vi "NewNearestNeighbor.vi"(4 "w":dbl=inf format="%#_13g", 6 "index":i32, 9 "p":dbl[](array[numeric]), 10 "q":dbl[](array[numeric]), 11 "KD-Tree":T1) -> (2 "Nearest":dbl[](array[numeric]))   [LabVIEW 2018]
uses:
  KD-Tree.ctl
  Node.ctl
  <vilib>/Analysis/_algsub.llb/Real Vector Norm.vi
  <vilib>/Analysis/NI_AALPro.lvlib
panel:
  out "Elapsed Time (s)":dbl
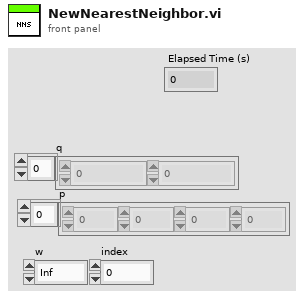
[diagram p1: front panel]
types:
  T1 = typedef "KD-Tree.ctl" = T2[]
  T2 = typedef "Node.ctl" = cluster{"axis":enum16{"null", "x", "y"}, "value":dbl, "left":dbl, "right":dbl, "Point":dbl[]}
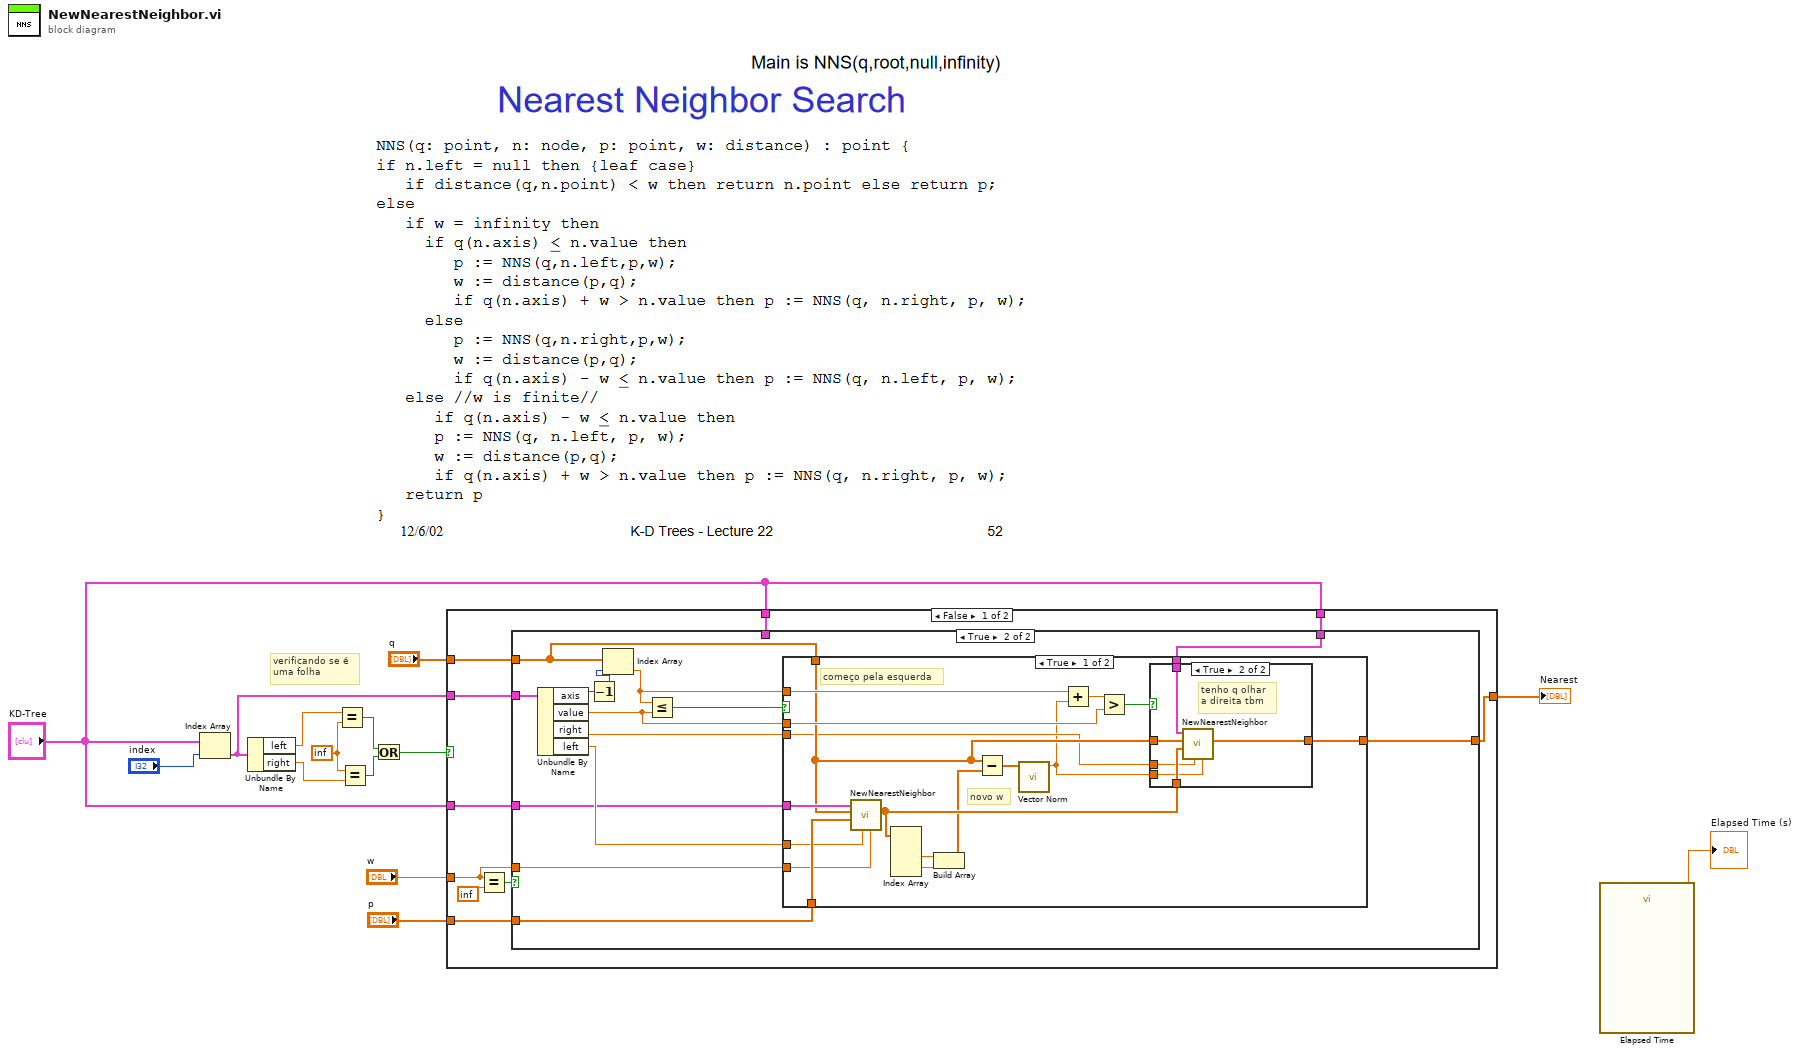
[diagram p0: block diagram]
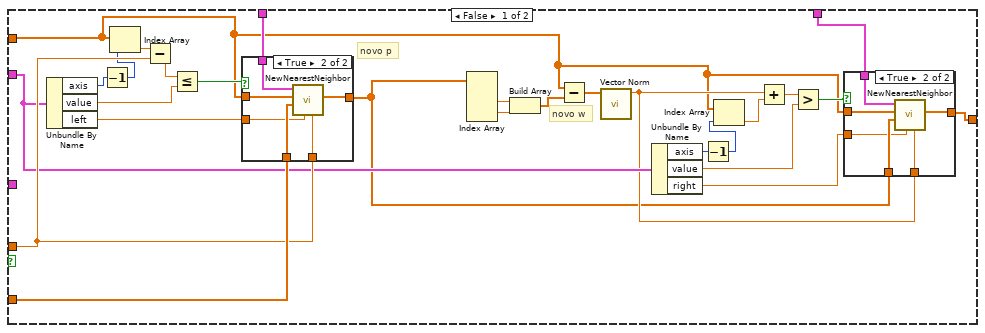
[diagram p2: hidden frame]
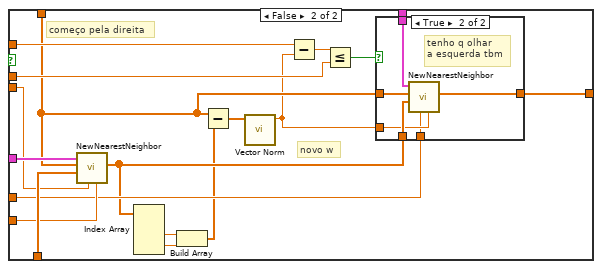
[diagram p6: hidden frame]
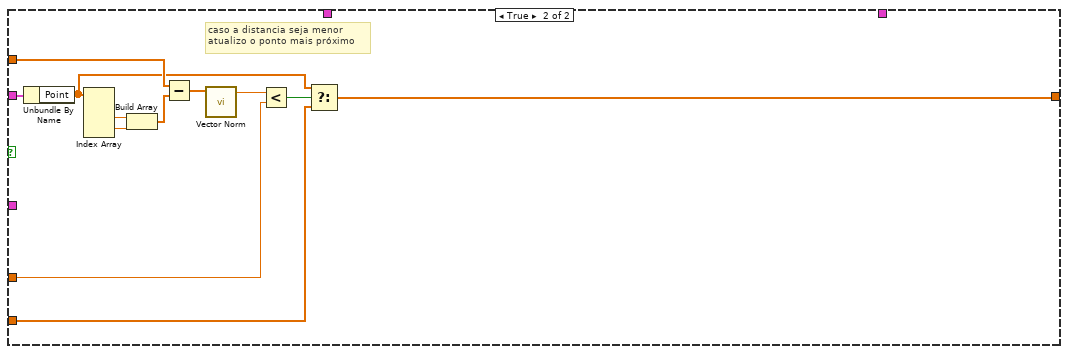
[diagram p8: hidden frame]
diagram:
  w13 = inf
  # "verificando se é \numa folha"
  n1 = Index Array(array="KD-Tree", index="index") -> (element=w7:T2)
  n2 = Unbundle By Name(w7) -> ("left"=w11:dbl, "right"=w12:dbl)
  n3 = Equal?(x=w11, y=w13) -> (x = y?=w9:bool)
  n4 = Equal?(x=w13, y=w12) -> (x = y?=w10:bool)
  n5 = Or(x=w9, y=w10) -> (x .or. y?=w8:bool)
  n6 = case shown="False" w8 {
    tunnel: w7 -> [w22 w141]
    tunnel: "q" -> [w21 w138]
    tunnel: "w" -> [w18 w135]
    tunnel: "p" -> [w19 w133]
    tunnel: [w16 w132] -> w3
    tunnel: "KD-Tree" -> [w20 _]
    tunnel: "KD-Tree" -> [w17 _]
    tunnel: "KD-Tree" -> [w15 _]
    frame False {
      n7 = Equal?(x=w18, y=inf) -> (x = y?=w24:bool)
      n8 = case shown="True" w24 {
        tunnel: w22 -> [w42 w79]
        tunnel: w21 -> [w33 w77]
        tunnel: w20 -> [_ w70]
        tunnel: w19 -> [w46 w76]
        tunnel: w18 -> [w44 w75]
        tunnel: w17 -> [w34 w69]
        tunnel: [w37 w68] -> w16
        tunnel: w15 -> [w47 _]
        frame False {
          # "novo p"
          # "novo w"
          n9 = Unbundle By Name(w42) -> ("axis"=w32:enum16{"null", "x", "y"}, "value"=w49:dbl, "left"=w45:dbl)
          n10 = Decrement(x=w32) -> (x-1=w31:enum16{"null", "x", "y"})
          n11 = Index Array(array=w33, index=w31) -> (element=w51:dbl)
          n12 = Subtract(x=w51, y=w44) -> (x-y=w50:dbl)
          n13 = Less Or Equal?(x=w50, y=w49) -> (x <= y?=w48:bool)
          n14 = case shown="True" w48 {
            tunnel: w47 -> [_ w65]
            tunnel: w33 -> [_ w64]
            tunnel: w46 -> [w59 w63]
            tunnel: w45 -> [_ w62]
            tunnel: w44 -> [_ w61]
            tunnel: [w59 w60] -> w26
            frame False {
            }
            frame True {
              n15 = call "NewNearestNeighbor.vi"("w"=w61, "index"=w62, "p"=w63, "q"=w64, "KD-Tree"=w65) -> ("Nearest"=w60:dbl[])  [unwired: 6 in]
            }
          }
          n16 = Index Array(array=w26) -> (element #2=w28:dbl, element #3=w27:dbl)  [unwired: 4 in, 2 out]
          n17 = Build Array(w28, w27) -> (w25:dbl[])
          n18 = Subtract(x=w33, y=w25) -> (x-y=w43:dbl[])
          n19 = call-poly <vilib>:"Vector Norm.vi"("Input Vector"=w43) -> ("norm"=w35:dbl)  [unwired: 9 in, 1 out]
          n20 = Unbundle By Name(w42) -> ("axis"=w30:enum16{"null", "x", "y"}, "value"=w39:dbl, "right"=w36:dbl)
          n21 = Decrement(x=w30) -> (x-1=w29:enum16{"null", "x", "y"})
          n22 = Index Array(array=w33, index=w29) -> (element=w41:dbl)
          n23 = Add(x=w35, y=w41) -> (x+y=w40:dbl)
          n24 = Greater?(x=w40, y=w39) -> (0:w38:bool)
          n25 = case shown="True" w38 {
            tunnel: w34 -> [_ w58]
            tunnel: w33 -> [_ w57]
            tunnel: w26 -> [w52 w56]
            tunnel: w36 -> [_ w55]
            tunnel: w35 -> [_ w54]
            tunnel: [w52 w53] -> w37
            frame False {
            }
            frame True {
              n26 = call "NewNearestNeighbor.vi"("w"=w54, "index"=w55, "p"=w56, "q"=w57, "KD-Tree"=w58) -> ("Nearest"=w53:dbl[])  [unwired: 6 in]
            }
          }
        }
        frame True {
          n27 = Unbundle By Name(w79) -> ("axis"=w67:enum16{"null", "x", "y"}, "value"=w71:dbl, "right"=w73:dbl, "left"=w74:dbl)
          n28 = Decrement(x=w67) -> (x-1=w66:enum16{"null", "x", "y"})
          n29 = Index Array(array=w77, index=w66) -> (element=w72:dbl)
          n30 = Less Or Equal?(x=w72, y=w71) -> (x <= y?=w78:bool)
          n31 = case shown="True" w78 {
            tunnel: w70 -> [w89 w115]
            tunnel: w77 -> [w87 w113]
            tunnel: w76 -> [w97 w122]
            tunnel: w74 -> [w96 w109]
            tunnel: w75 -> [w95 w121]
            tunnel: w73 -> [w86 w110]
            tunnel: w72 -> [w93 w119]
            tunnel: w71 -> [w91 w117]
            tunnel: w69 -> [w88 w114]
            tunnel: [w84 w111] -> w68
            frame True {
              # "novo w"
              # "começo pela esquerda"
              n32 = call "NewNearestNeighbor.vi"("w"=w95, "index"=w96, "p"=w97, "q"=w87, "KD-Tree"=w89) -> ("Nearest"=w81:dbl[])  [unwired: 6 in]
              n33 = Index Array(array=w81) -> (element #2=w83:dbl, element #3=w82:dbl)  [unwired: 4 in, 2 out]
              n34 = Build Array(w83, w82) -> (w80:dbl[])
              n35 = Subtract(x=w87, y=w80) -> (x-y=w94:dbl[])
              n36 = call-poly <vilib>:"Vector Norm.vi"("Input Vector"=w94) -> ("norm"=w85:dbl)  [unwired: 9 in, 1 out]
              n37 = Add(x=w93, y=w85) -> (x+y=w92:dbl)
              n38 = Greater?(x=w92, y=w91) -> (0:w90:bool)
              n39 = case shown="True" w90 {
                tunnel: w88 -> [_ w104]
                tunnel: w87 -> [_ w103]
                tunnel: w81 -> [w98 w102]
                tunnel: w86 -> [_ w101]
                tunnel: w85 -> [_ w100]
                tunnel: [w98 w99] -> w84
                frame False {
                  # "n é necessário \nolhar a direita"
                }
                frame True {
                  # "tenho q olhar \na direita tbm"
                  n40 = call "NewNearestNeighbor.vi"("w"=w100, "index"=w101, "p"=w102, "q"=w103, "KD-Tree"=w104) -> ("Nearest"=w99:dbl[])  [unwired: 6 in]
                }
              }
            }
            frame False {
              # "novo w"
              # "começo pela direita"
              n41 = call "NewNearestNeighbor.vi"("w"=w121, "index"=w110, "p"=w122, "q"=w113, "KD-Tree"=w115) -> ("Nearest"=w106:dbl[])  [unwired: 6 in]
              n42 = Index Array(array=w106) -> (element #2=w108:dbl, element #3=w107:dbl)  [unwired: 4 in, 2 out]
              n43 = Build Array(w108, w107) -> (w105:dbl[])
              n44 = Subtract(x=w113, y=w105) -> (x-y=w120:dbl[])
              n45 = call-poly <vilib>:"Vector Norm.vi"("Input Vector"=w120) -> ("norm"=w112:dbl)  [unwired: 9 in, 1 out]
              n46 = Subtract(x=w119, y=w112) -> (x-y=w118:dbl)
              n47 = Less Or Equal?(x=w118, y=w117) -> (x <= y?=w116:bool)
              n48 = case shown="True" w116 {
                tunnel: w114 -> [_ w129]
                tunnel: w113 -> [_ w128]
                tunnel: w106 -> [w123 w127]
                tunnel: w112 -> [_ w126]
                tunnel: [w123 w125] -> w111
                tunnel: w109 -> [_ w124]
                frame False {
                  # "n é necessário \nolhar a esquerda"
                }
                frame True {
                  # "tenho q olhar \na esquerda tbm"
                  n49 = call "NewNearestNeighbor.vi"("w"=w126, "index"=w124, "p"=w127, "q"=w128, "KD-Tree"=w129) -> ("Nearest"=w125:dbl[])  [unwired: 6 in]
                }
              }
            }
          }
        }
      }
    }
    frame True {
      # "caso a distancia seja menor \natualizo o ponto mais próximo"
      n50 = Unbundle By Name(w141) -> ("Point"=w131:dbl[])
      n51 = Index Array(array=w131) -> (element #2=w140:dbl, element #3=w139:dbl)  [unwired: 4 in, 2 out]
      n52 = Build Array(w140, w139) -> (w130:dbl[])
      n53 = Subtract(x=w138, y=w130) -> (x-y=w137:dbl[])
      n54 = call-poly <vilib>:"Vector Norm.vi"("Input Vector"=w137) -> ("norm"=w136:dbl)  [unwired: 9 in, 1 out]
      n55 = Less?(x=w136, y=w135) -> (x < y?=w134:bool)
      n56 = Select(t=w131, s=w134, f=w133) -> (s? t:f=w132:dbl[])
    }
  }
  "Nearest" <- w3
  n57 = call "Elapsed Time"() -> ("Elapsed Time (s)"=→"Elapsed Time (s)":dbl)  [unwired: 12 in, 7 out]
